vi "TinyPackets.vi"(2 "Max Size":i32=500, 3 "Translate":enum16{"None", "Tiny", "URAPI"}(ring), 4 "URAPI Script":T1={"Script"="count0=0\n//while0 forever\nforever:\ncount0=count0+1\nD!0=count0\ncount0+=1\ngoto forever\n", "Whiles"=[], "Ifs"=[], "Supress Err"=TRUE, "Errors"=""}) -> (1 "Script Packets":string[](array[string]))   [LabVIEW 2012]
uses:
  <userlib>/BotSpeak/VIs/Direct/URAPI_Control.ctl
  <userlib>/BotSpeak/VIs/SubVIs/BotSpeak_Globals.vi
panel:
  out "script":string="SET count0,0\n\nADD count0,1\nDIO 0,count0\nADD count0,1\ngoto 2\n"
  out "# chars":i32=28
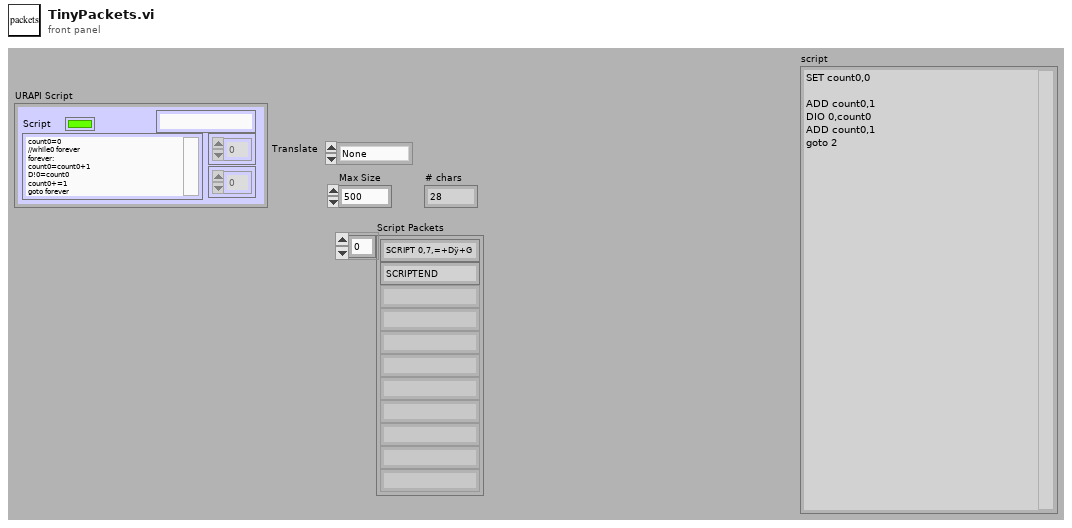
[diagram p1: front panel]
types:
  T1 = typedef "URAPI_Control.ctl" = cluster{"Script":string, "Whiles":u8[], "Ifs":u8[], "Supress Err":bool, "Errors":string}
  T2 = cluster{"Sent":string, "reply":string, "reply 2":string}[]
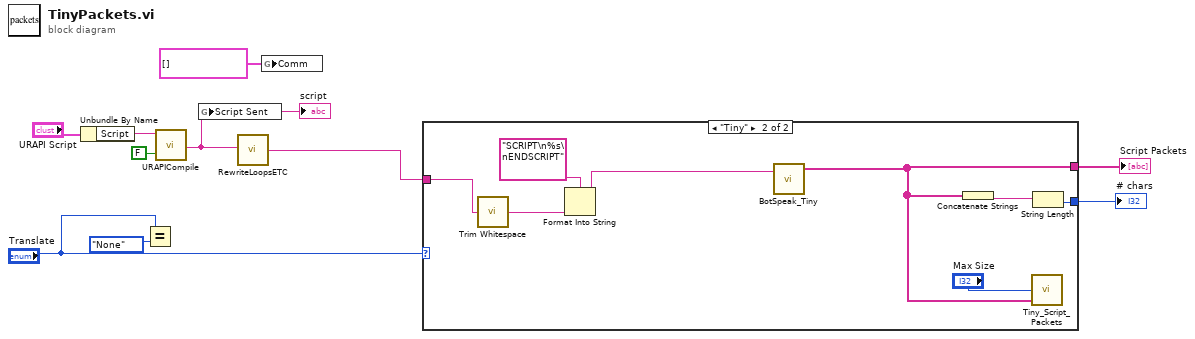
[diagram p0: block diagram]
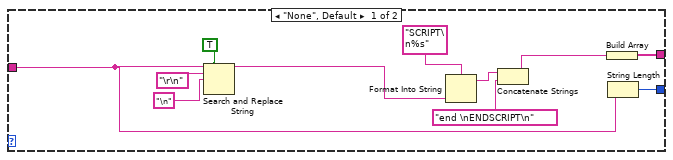
[diagram p2: hidden frame]
diagram:
  n1 = Unbundle By Name("URAPI Script") -> ("Script"=w7:string)
  n2 = Equal?(x="Translate", y=enum16{"None", "Tiny", "URAPI"}."None") -> ()  [unwired: 1 out]
  n3 = call <userlib>:"URAPICompile.vi"("Comments?"=FALSE, "Script"=w7) -> ("trimmed script"=w2:string)
  "script" <- w2
  n4 = global write "BotSpeak_Globals.vi" "Script Sent"(w2) -> ()
  n5 = call <userlib>:"RewriteLoopsETC.vi"("URAPI in"=w2) -> ("URAPI out"=w1:string)  [unwired: 1 in]
  n6 = global write "BotSpeak_Globals.vi" "Comm"(T2 [] ("Comm")) -> ()
  n7 = case shown="\"Tiny\"" "Translate" {
    tunnel: [w20 w25] -> w9
    tunnel: [w21 w23] -> w8
    tunnel: w1 -> [w11 w27]
    frame "None", Default {
      n8 = Search and Replace String(replace all?=TRUE ("replace all? (F)"), input string=w11, search string="\r\n", replace string="\n" ("search string")) -> (result string=w16:string)  [unwired: 4 in, 3 out]
      n9 = Format Into String(format string="SCRIPT\n%s" ("command"), w16) -> (resulting string=w14:string)  [unwired: 2 in, 1 out]
      n10 = Concatenate Strings(w14, "end \nENDSCRIPT\n" ("search string")) -> (w13:string)
      n11 = Build Array(w13) -> (w20:string[])
      n12 = String Length(string=w11) -> (length=w21:i32)
    }
    frame "Tiny" {
      n13 = call <vilib>:"Trim Whitespace.vi"("string"=w27) -> ("trimmed string"=w26:string)  [unwired: 1 in]
      n14 = Format Into String(format string="SCRIPT\n%s\nENDSCRIPT" ("command"), w26) -> (resulting string=w28:string)  [unwired: 2 in, 1 out]
      n15 = call <userlib>:"BotSpeak_Tiny.vi"("URAPI"=w28) -> ("Tiny Lines"=w25:string[])  [unwired: 1 in, 2 out]
      n16 = Concatenate Strings(w25) -> (w24:string)
      n17 = call <userlib>:"Tiny_Script_Packets.vi"("Lines in"=w25, "Max Size"="Max Size") -> ()  [unwired: 1 in, 2 out]
      n18 = String Length(string=w24) -> (length=w23:i32)
    }
  }
  "Script Packets" <- w9
  "# chars" <- w8
